vi "PAN_Translate.vi"(0 "command in":string, 1 "app ID":string, 5 "Table":string[][](table), 11 "error in (no error)":errorcluster) -> (4 "command out":string, 15 "error out":errorcluster)   [LabVIEW 2016]
panel:
  # "commmand"
  # "hardware"
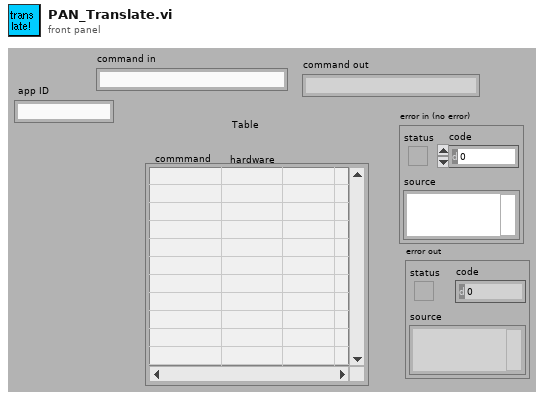
[diagram p1: front panel]
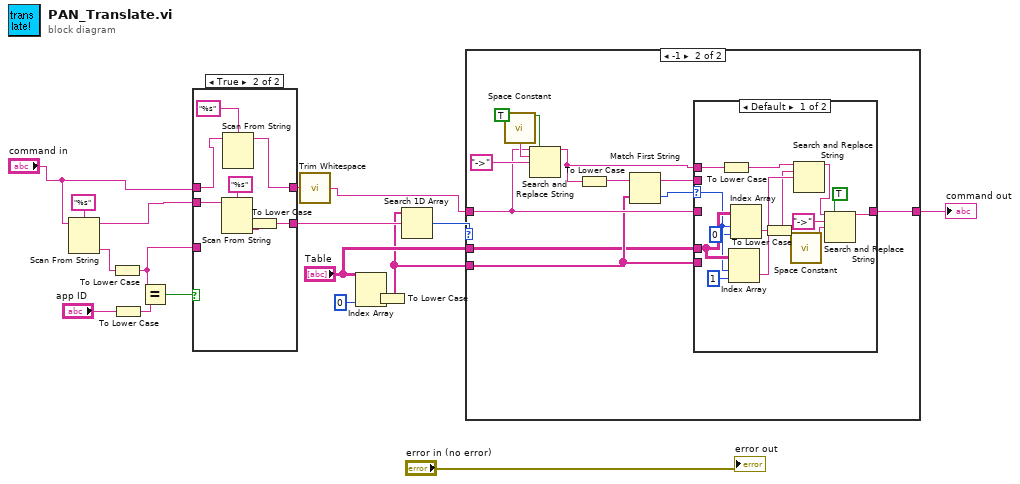
[diagram p0: block diagram]
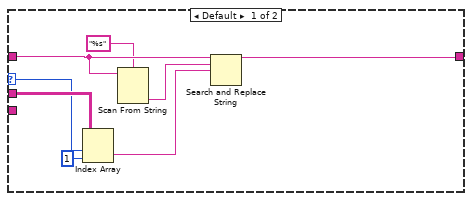
[diagram p3: hidden frame]
diagram:
  n1 = Scan From String(format string="%s", input string="command in") -> (remaining string=w3:string, output 1=w6:string)  [unwired: 2 in, 3 out]
  n2 = To Lower Case(string=w6) -> (all lower case string=w4:string)
  n3 = To Lower Case(string="app ID") -> (all lower case string=w9:string)
  n4 = Equal?(x=w4, y=w9) -> (x = y?=w8:bool)
  n5 = case shown="True" w8 {
    tunnel: "command in" -> [w20 w23]
    tunnel: [w20 w21] -> w7
    tunnel: w4 -> [w19 _]
    tunnel: [w19 w25] -> w5
    tunnel: w3 -> [_ w24]
    frame False {
    }
    frame True {
      n6 = Scan From String(format string="%s", input string=w24) -> (output 1=w26:string)  [unwired: 2 in, 4 out]
      n7 = Scan From String(format string="%s", input string=w23) -> (remaining string=w21:string)  [unwired: 2 in, 4 out]
      n8 = To Lower Case(string=w26) -> (all lower case string=w25:string)
    }
  }
  n9 = call <vilib>:"Trim Whitespace.vi"("string"=w7) -> ("trimmed string"=w12:string)  [unwired: 1 in]
  n10 = Index Array(array="Table", index (col)=0 ("disabled index (col)")) -> (element=w13:string[])  [unwired: 1 in]
  n11 = To Lower Case(string=w13) -> (all lower case string=w2:string[])
  n12 = Search 1D Array(1D array=w2, element=w5) -> (index of element=w17:i32)  [unwired: 1 in]
  n13 = case shown="-1" w17 {
    selector: w17 -> [w34 _]
    tunnel: w12 -> [w32 w44]
    tunnel: [w28 w43] -> w16
    tunnel: "Table" -> [w35 w39]
    tunnel: w2 -> [_ w40]
    frame Default {
      n14 = Index Array(array=w35, index (row)=w34, index (col)=1 ("disabled index (col)")) -> (element=w29:string)
      n15 = Scan From String(format string="%s", input string=w32) -> (output 1=w30:string)  [unwired: 2 in, 4 out]
      n16 = Search and Replace String(input string=w32, search string=w30, replace string=w29) -> (result string=w28:string)  [unwired: 1 in, 7 out]
    }
    frame -1 {
      n17 = call <vilib>:"Space Constant.vi"() -> ("String"=w46:string)
      n18 = Search and Replace String(replace all?=TRUE ("replace all? (F)"), input string=w44, search string=w46, replace string="->" ("replace string (\"\")")) -> (result string=w36:string)  [unwired: 1 in, 6 out]
      n19 = To Lower Case(string=w36) -> (all lower case string=w38:string)
      n20 = Match First String(2:w40, 3:w38) -> (0:w42:i32, 1:w41:string)
      n21 = case shown="Default" w42 {
        selector: w42 -> [w58 _]
        tunnel: w44 -> [_ w61]
        tunnel: [w50 w61] -> w43
        tunnel: w41 -> [_ _]
        tunnel: w40 -> [_ _]
        tunnel: w39 -> [w59 _]
        tunnel: w36 -> [w56 _]
        frame Default {
          n22 = To Lower Case(string=w56) -> (all lower case string=w48:string)
          n23 = Index Array(array=w59, index (row)=w58, index (col)=1 ("disabled index (col)")) -> (element=w54:string)
          n24 = Index Array(array=w59, index (row)=w58, index (col)=0 ("disabled index (col)")) -> (element=w55:string)
          n25 = To Lower Case(string=w55) -> (all lower case string=w47:string)
          n26 = call <vilib>:"Space Constant.vi"() -> ("String"=w51:string)
          n27 = Search and Replace String(input string=w48, search string=w47, replace string=w54) -> (result string=w53:string)  [unwired: 1 in, 7 out]
          n28 = Search and Replace String(replace all?=TRUE ("replace all? (F)"), input string=w53, search string="->", replace string=w51) -> (result string=w50:string)  [unwired: 1 in, 6 out]
        }
        frame -1 {
        }
      }
    }
  }
  "command out" <- w16
  "error out" <- "error in (no error)"
